vi "Auto Match.vi"() -> ()   [LabVIEW 2022 SP3]
panel:
  out "Number of iterations":i32
  out "Current Number":u32
  in  "Number to match":u32=50 min=1 max=1000 step=1
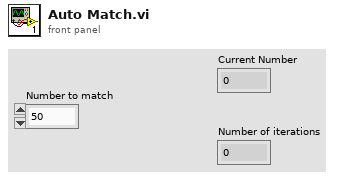
[diagram p1: front panel]
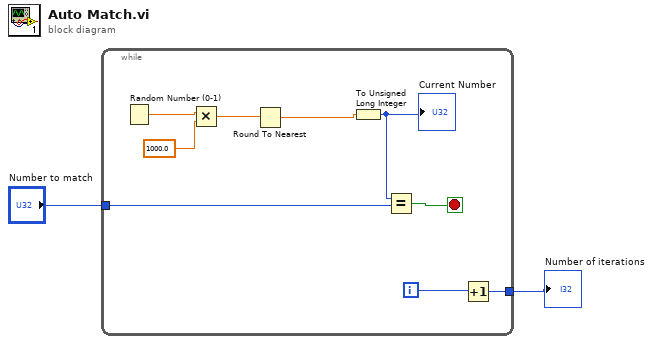
[diagram p0: block diagram]
diagram:
  n1 = while {
    tunnel: "Number to match" -> [w8]
    tunnel: [w4] -> w1
    i -> [w5]
    stop <- w6 stop-if-true
    n2 = Random Number (0-1)() -> (number: 0 to 1=w11:dbl)
    n3 = Multiply(x=w11, y=1000.0) -> (x*y=w9:dbl)
    n4 = Round To Nearest(number=w9) -> (nearest integer value=w7:dbl)
    n5 = To Unsigned Long Integer(number=w7) -> (unsigned 32bit integer=w3:u32)
    "Current Number" <- w3
    n6 = Equal?(x=w3, y=w8) -> (x = y?=w6:bool)
    n7 = Increment(x=w5) -> (x+1=w4:i32)
  }
  "Number of iterations" <- w1
